vi "PPS_TRAJECTORY_EXECUTE_REL.vi"(8 "Init":bool, 10 "End Relative\nOrientation Deg":dbl, 11 "Gyro Heading\nRAD":dbl) -> (0 "AtReference":bool, 3 "Chassis Velocity Target SI":T3 {"vOmega" format="%10.3f"; "vY" format="%10.3f"; "vX" format="%10.3f"})   [LabVIEW 2019]
uses:
  <vilib>/Rock Robotics/WPI/ThirdParty/JAS_Junk/TrajLib/Trajectory_Library.lvlib
  CHS_TRAJECTORY_GLOBALS.vi
  <vilib>/Rock Robotics/WPI/ThirdParty/MJansen/PathPlanner/PathPlanner24.lvlib
  <vilib>/Rock Robotics/WPI/ThirdParty/JAS_Junk/TrajLib/TypeDef/CHASSIS_SPEEDS.ctl
  <vilib>/Rock Robotics/WPI/ThirdParty/ChoreoLib/TypeDef/ChoreoTrajectoryState.ctl
  <vilib>/Rock Robotics/WPI/ThirdParty/ChoreoLib/ChoreoLib.lvlib
  <vilib>/Rock Robotics/WPI/ThirdParty/ChoreoLib/TypeDef/ChoreoTrajectory.ctl
panel:
  out "ChoreoTrajectory":T1
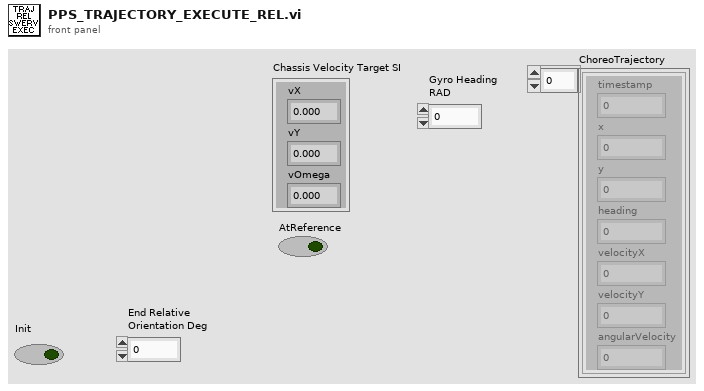
[diagram p1: front panel]
types:
  T1 = typedef "ChoreoLib.lvlib/ChoreoTrajectory.ctl" = T2[]
  T2 = typedef "ChoreoLib.lvlib/ChoreoTrajectoryState.ctl" = cluster{"timestamp":dbl, "x":dbl, "y":dbl, "heading":dbl, "velocityX":dbl, "velocityY":dbl, "angularVelocity":dbl}
  T3 = typedef "Trajectory_Library.lvlib/CHASSIS_SPEEDS.ctl" = cluster{"vX":dbl, "vY":dbl, "vOmega":dbl}
  T4 = typedef "Trajectory_Library.lvlib/SWERVE_DRIVE_KINEMATICS.ctl" = cluster{"NumModules":i32, "InverseKinematics":T5, "ForwardKinematics":T5, "Modules":T6[], "PrevCoR":T6, "SavedModuleStates":T7[]}
  T5 = typedef "NI_Matrix.lvlib/RealMatrix.ctl" = dbl[][]
  T6 = typedef "Trajectory_Library.lvlib/TRANSLATION2D.ctl" = cluster{"X":dbl, "Y":dbl}
  T7 = typedef "Trajectory_Library.lvlib/SWERVE_DRIVE_MODULE_STATE.ctl" = cluster{"Speed":dbl, "Angle":T8}
  T8 = typedef "Trajectory_Library.lvlib/ROTATION2D.ctl" = cluster{"VALUE":dbl, "COS":dbl, "SIN":dbl}
  T9 = typedef "Trajectory_Library.lvlib/SWERVE_DRIVE_MODULE_POSITION.ctl" = cluster{"Distance":dbl, "Angle":T8, "P":bool}
  T10 = typedef "Trajectory_Library.lvlib/POSE2D.ctl" = cluster{"TRANSLATION":T6, "ROTATION":T8}
  T11 = typedef "PathPlanner24.lvlib/PathPlannerTrajectoryState.ctl" = cluster{"TimeSeconds":dbl, "VelocityMPS":dbl, "AccerationMpsSq":dbl, "HeadingAngularVelRadPerSec":dbl, "PositionMeters":T6, "Heading":T8, "TargetHolonomicRotation":T8, "CurvatureRadPerMeter":dbl, "PathPlannerConstraints":T12, "DeltaPos":dbl}
  T12 = typedef "PathPlanner24.lvlib/PathPlannerPathConstraints.ctl" = cluster{"MaxVelocityMps;":dbl, "MaxAccelerationMpsSq;":dbl, "MaxAngularVelRadPsEc;":dbl, "MaxAngularAccRadPSecSq":dbl, "Exists":bool}
  T13 = typedef "Trajectory_Library.lvlib/PID_TUNING.ctl" = cluster{"Kp":dbl, "Ki":dbl, "Kd":dbl, "MaximumIntegral":dbl, "MinimumIntegral":dbl}
  T14 = typedef "Trajectory_Library.lvlib/PROFILED_PID_CONTROLLER.ctl" = cluster{"Controller":T15, "Goal":T16, "Setpoint":T16, "Constraint":T17}
  T15 = typedef "Trajectory_Library.lvlib/PID_CONTROLLER.ctl" = cluster{"Kp":dbl, "Ki":dbl, "Kd":dbl, "Period":dbl, "Max_Integral":dbl, "Min_Integral":dbl, "Max_Input":dbl, "Min_Input":dbl, "Continuous":bool, "PositionError":dbl, "VelocityError":dbl, "PrevError":dbl, "TotalError":dbl, "PositionTolerance":dbl, "VelocityTolerance":dbl, "SetPoint":dbl, "Kf":dbl, "Prev_Deriv":dbl, "Prev_Deriv 2":dbl, "DerivativeFilter":bool, "Min_Output":dbl, "Max_Output":dbl, "Prev_F_P":dbl, "Prev_F_P_2":dbl, "AntiWindupActive":bool, "Measurement":dbl}
  T16 = typedef "Trajectory_Library.lvlib/TRAPEZOID_PROFILE_STATE.ctl" = cluster{"Position":dbl, "Velocity":dbl}
  T17 = typedef "Trajectory_Library.lvlib/TRAPEZOID_PROFILE_CONSTRAINT.ctl" = cluster{"MaxVelocity":dbl, "MaxAcceleration":dbl}
  T18 = typedef "PathPlanner24.lvlib/PathPlannerCtrlHolConfig.ctl" = cluster{"HOLONOMIC_CTRL_PACK_TUNING":T19, "Max Wheel Speed M/S":dbl, "Tolerance SI":T10, "Drive Base Radius M":dbl}
  T19 = typedef "Trajectory_Library.lvlib/HOLONOMIC_PACK_TUNING.ctl" = cluster{"X PID Tuning":T13, "Y PID Tuning":T13, "thetaProfiledPID_CTRL":T14}
  T20 = typedef "Trajectory_Library.lvlib/HOLONOMIC_DRV_CTRL.ctl" = cluster{"poseTolerance":T10, "poseError":T10, "Enabled":bool, "PID_xCtrl":T15, "PID_yCtrl":T15, "PROF_PID_thetaCtrl":T14, "RotationError":T8, "FirstRun":bool}
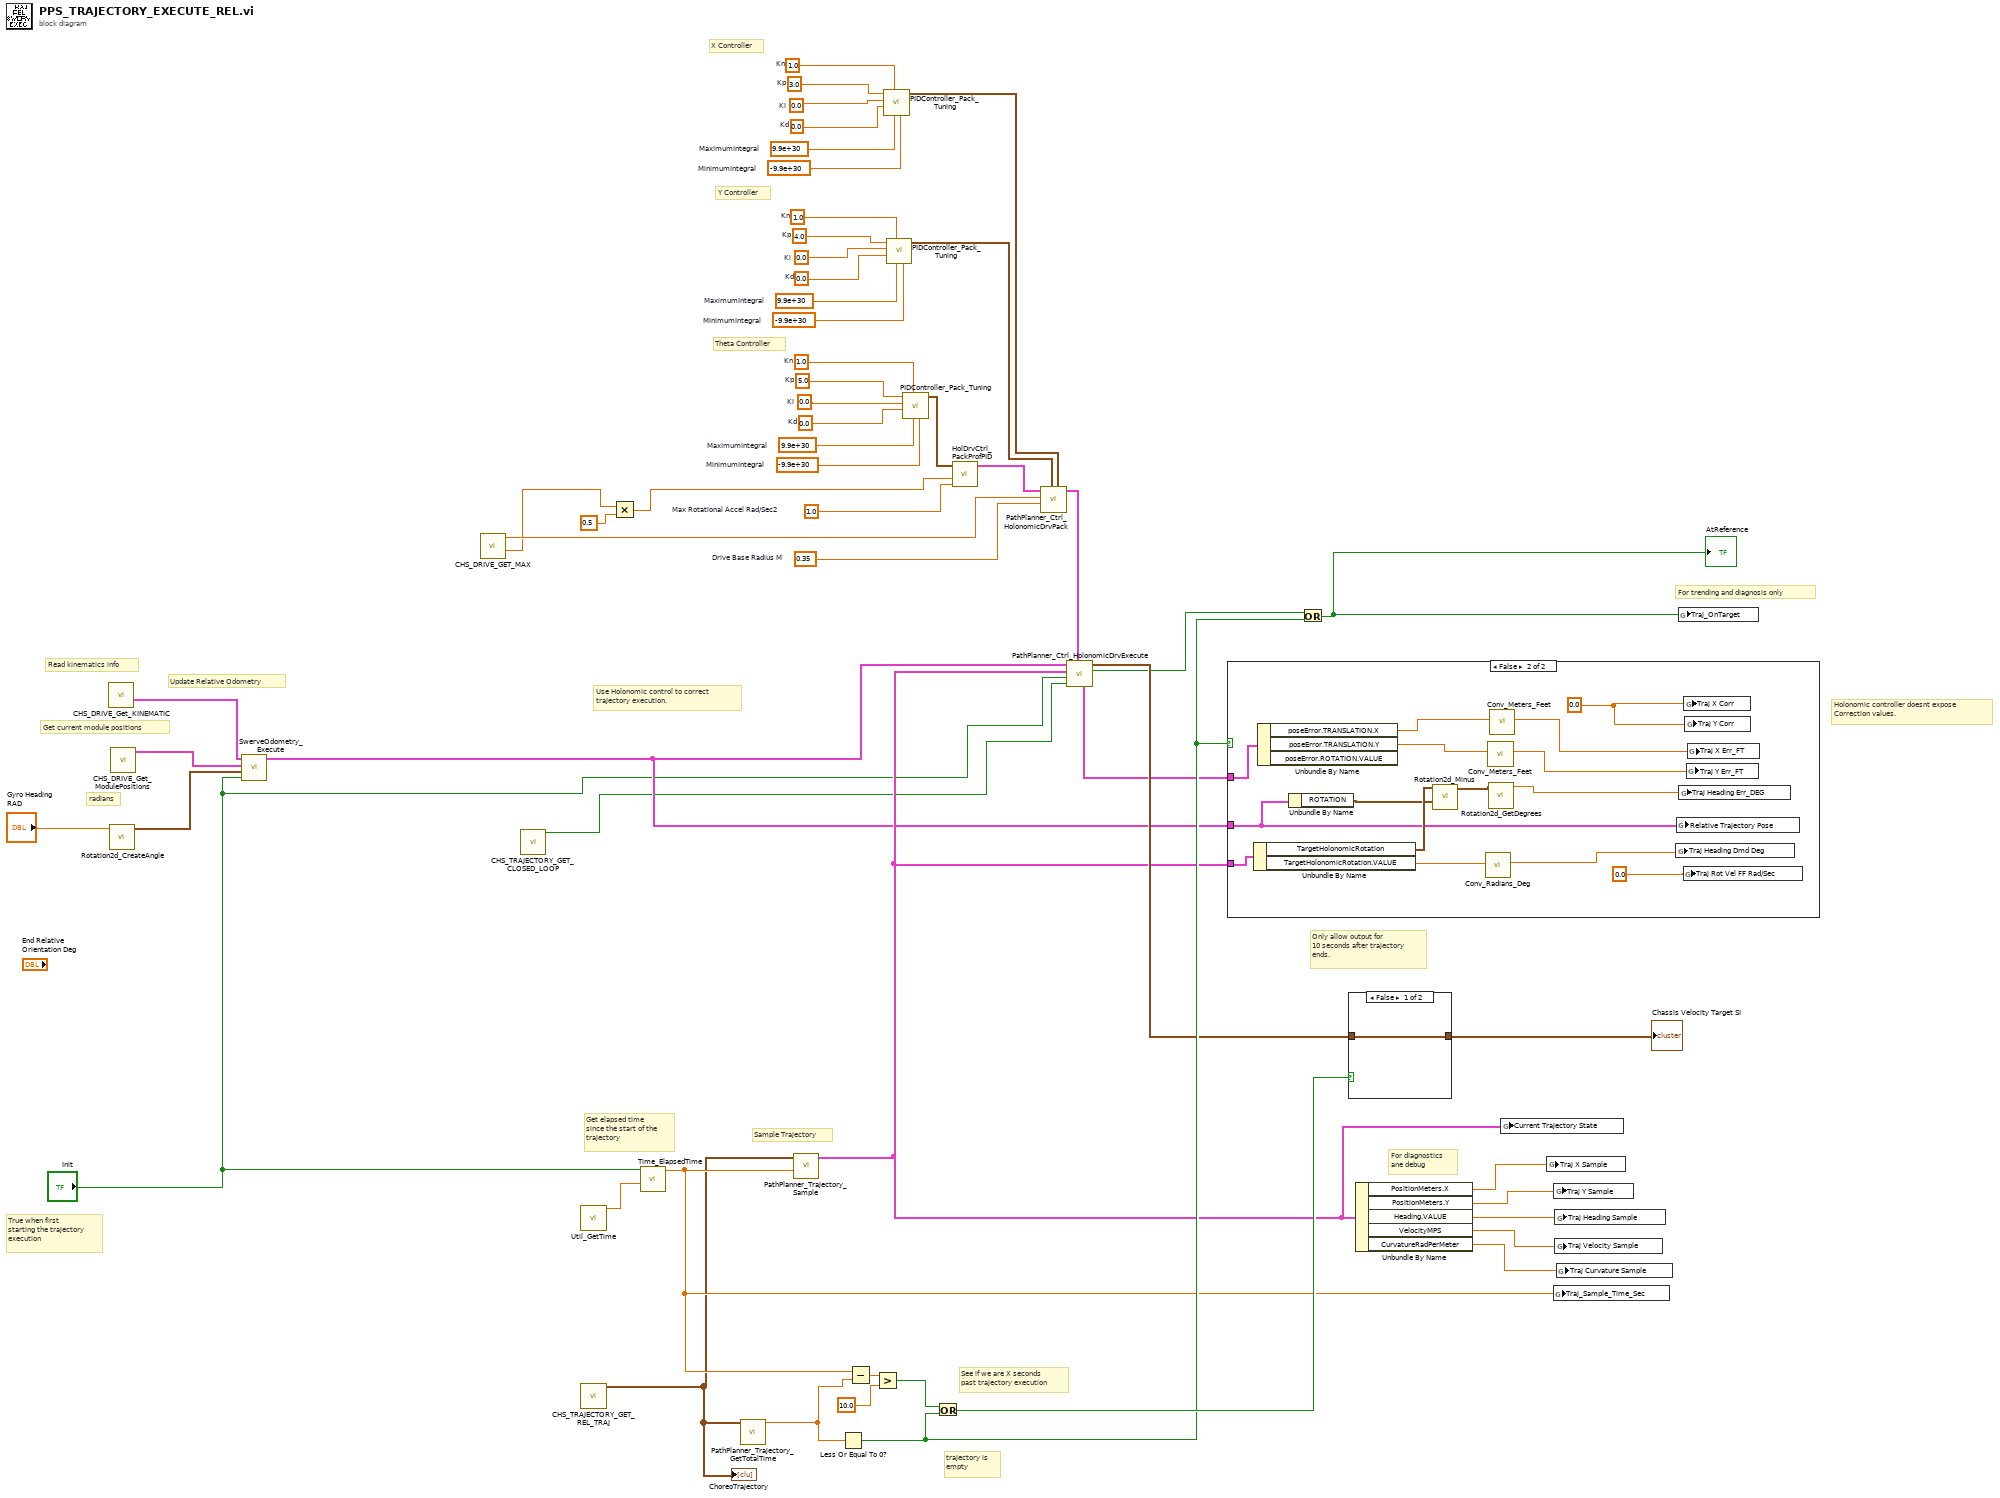
[diagram p0: block diagram]
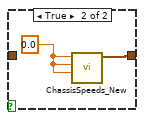
[diagram p3: hidden frame]
diagram:
  w32 = 0.35  # Drive Base Radius M
  w24 = 1.0  # Kn
  w21 = 5.0  # Kp
  w12 = 0.0  # Ki
  w11 = 0.0  # Kd
  w10 = 9.9e+30  # MaximumIntegral
  w9 = -9.9e+30  # MinimumIntegral
  w26 = 1.0  # Kn
  w23 = 3.0  # Kp
  w20 = 0.0  # Ki
  w19 = 0.0  # Kd
  w18 = 9.9e+30  # MaximumIntegral
  w17 = -9.9e+30  # MinimumIntegral
  w25 = 1.0  # Kn
  w22 = 4.0  # Kp
  w16 = 0.0  # Ki
  w15 = 0.0  # Kd
  w14 = 9.9e+30  # MaximumIntegral
  w13 = -9.9e+30  # MinimumIntegral
  w27 = 1.0  # Max Rotational Accel Rad/Sec2
  # "Theta Controller"
  # "Y Controller"
  # "X Controller"
  # "Get current module positions"
  # "Update Relative Odometry"
  # "Read kinematics info"
  # "radians"
  # "trajectory is \nempty"
  # "True when first\nstarting the trajectory\nexecution"
  # "Get elapsed time\nsince the start of the\ntrajectory"
  # "Holonomic controller doesnt expose\nCorrection values."
  # "Use Holonomic control to correct\ntrajectory execution."
  # "For trending and diagnosis only"
  # "For diagnostics\nane debug"
  # "Sample Trajectory"
  # "See if we are X seconds \npast trajectory execution"
  # "Only allow output for\n10 seconds after trajectory\nends."
  n1 = call "CHS_DRIVE_Get_KINEMATIC.vi"() -> ("out SWERVE_DRIVE_KINEMATICS"=w35:T4)  [unwired: 11 in]
  n2 = call <vilib>:"Rotation2d_CreateAngle.vi"("Angle"="Gyro Heading\nRAD") -> ("ROTATION"=w37:T8)  [unwired: 10 in]
  n3 = call "CHS_DRIVE_Get_ModulePositions.vi"() -> ("Swerve Module Positions"=w36:T9[])  [unwired: 11 in]
  n4 = call <vilib>:"SwerveOdometry_Execute.vi"("Init"="Init", "Rotation"=w37, "Swerve Module Positions"=w36, "SWERVE_DRIVE_KINEMATICS"=w35) -> ("Current Pose"=w34:T10)  [unwired: 5 in, 2 out]
  n5 = call "CHS_DRIVE_GET_MAX.vi"() -> ("Max Rotational Vel (Rad/Sec)"=w2:dbl, "Max Wheel Vel (Meter/Sec)"=w6:dbl)  [unwired: 10 in]
  n6 = call "CHS_TRAJECTORY_GET_CLOSED_LOOP.vi"() -> ("AUTO_CLOSED_LOOP"=w4:bool)  [unwired: 11 in]
  n7 = call <vilib>:"Util_GetTime.vi"() -> ("FPGA_Time_Seconds"=w53:dbl)  [unwired: 9 in, 2 out]
  n8 = call "CHS_TRAJECTORY_GET_REL_TRAJ.vi"() -> ("Relative_Trajectory"=w38:T1)  [unwired: 11 in]
  "ChoreoTrajectory" <- w38
  n9 = Multiply(x=w2, y=0.5) -> (x*y=w1:dbl)
  n10 = call <vilib>:"Time_ElapsedTime.vi"("PassthroughTime_SEC"=w53, "Reset"="Init") -> ("Elapsed Time Sec"=w43:dbl)  [unwired: 9 in]
  n11 = call <vilib>:"PathPlanner_Trajectory_GetTotalTime.vi"("PathPlannerTrajectory"=w38) -> ("TotalTimeSeconds"=w40:dbl)  [unwired: 10 in]
  n12 = call <vilib>:"PathPlanner_Trajectory_Sample.vi"("Time"=w43, "PathPlannerTrajectory"=w38) -> ("PathPlannerState"=w39:T11)  [unwired: 9 in]
  n13 = Less Or Equal To 0?(x=w40) -> (x <= 0?=w44:bool)
  n14 = Subtract(x=w43, y=w40) -> (x-y=w56:dbl)
  n15 = Greater?(x=w56, y=10.0) -> (0:w47:bool)
  n16 = call <vilib>:"PIDController_Pack_Tuning.vi"("MinimumIntegral"=w17, "MaximumIntegral"=w18, "Kn"=w26, "Kd"=w19, "Ki"=w20, "Kp"=w23) -> ("PID Tuning"=w29:T13)  [unwired: 5 in]
  n17 = call <vilib>:"PIDController_Pack_Tuning.vi"("MinimumIntegral"=w13, "MaximumIntegral"=w14, "Kn"=w25, "Kd"=w15, "Ki"=w16, "Kp"=w22) -> ("PID Tuning"=w30:T13)  [unwired: 5 in]
  n18 = call <vilib>:"PIDController_Pack_Tuning.vi"("MinimumIntegral"=w9, "MaximumIntegral"=w10, "Kn"=w24, "Kd"=w11, "Ki"=w12, "Kp"=w21) -> ("PID Tuning"=w28:T13)  [unwired: 5 in]
  n19 = Or(x=w47, y=w44) -> (x .or. y?=w46:bool)
  n20 = call <vilib>:"HolDrvCtrl_PackProfPID.vi"("Max Accel"=w27, "Max Speed"=w1, "Theta PID Tuning"=w28) -> ("Theta PID CONTROLLER"=w31:T14)  [unwired: 8 in]
  n21 = call <vilib>:"PathPlanner_Ctrl_HolonomicDrvPack.vi"("X PID Tuning"=w29, "Y PID Tuning"=w30, "Drive Base Radius M"=w32, "Max Wheel Speed M/S"=w6, "thetaProfiledPID_CTRL"=w31) -> ("PathPlanner_Ctrl_HolDrvConfig"=w8:T18)  [unwired: 6 in]
  n22 = call <vilib>:"PathPlanner_Ctrl_HolonomicDrvExecute.vi"("PathPlanner_Ctrl_HolDrvConfig"=w8, "Enabled"=w4, "Reset"="Init", "PathPlannerState"=w39, "Current Pose SI"=w34) -> ("At Reference"=w41:bool, "calcChassisSpeed"=w42:T3, "outHOLONOMIC_DRV_CTRL"=w7:T20)  [unwired: 3 in, 1 out]
  n23 = case shown="False" w44 {
    tunnel: w34 -> [_ w60]
    tunnel: w7 -> [_ w67]
    tunnel: w39 -> [_ w64]
    frame True {
    }
    frame False {
      w71 = 0.0 ("Y Corr")
      n24 = Unbundle By Name(w64) -> ("TargetHolonomicRotation"=w61:T8, "TargetHolonomicRotation.VALUE"=w63:dbl)
      n25 = Unbundle By Name(w67) -> ("poseError.TRANSLATION.X"=w66:dbl, "poseError.TRANSLATION.Y"=w65:dbl)  [unwired: 1 out]
      n26 = Unbundle By Name(w60) -> ("ROTATION"=w59:T8)
      n27 = call <vilib>:"Rotation2d_Minus.vi"("other ROTATION"=w59, "in ROTATION"=w61) -> ("out ROTATION"=w58:T8)  [unwired: 9 in]
      n28 = call <vilib>:"Conv_Radians_Deg.vi"("Radians"=w63) -> ("Degrees"=w62:dbl)  [unwired: 10 in]
      n29 = call <vilib>:"Conv_Meters_Feet.vi"("Meters"=w65) -> ("Feet"=w70:dbl)  [unwired: 10 in]
      n30 = call <vilib>:"Rotation2d_GetDegrees.vi"("in ROTATION"=w58) -> ("AngleDegrees"=w57:dbl)  [unwired: 10 in]
      n31 = call <vilib>:"Conv_Meters_Feet.vi"("Meters"=w66) -> ("Feet"=w69:dbl)  [unwired: 10 in]
      n32 = global write "CHS_TRAJECTORY_GLOBALS.vi" "Traj Heading Dmd Deg"(w62) -> ()
      n33 = global write "CHS_TRAJECTORY_GLOBALS.vi" "Relative Trajectory Pose"(w60) -> ()
      n34 = global write "CHS_TRAJECTORY_GLOBALS.vi" "Traj Heading Err_DEG"(w57) -> ()
      n35 = global write "CHS_TRAJECTORY_GLOBALS.vi" "Traj Rot Vel FF Rad/Sec"(0.0 ("Traj Heading Dmd Deg")) -> ()
      n36 = global write "CHS_TRAJECTORY_GLOBALS.vi" "Traj X Corr"(w71) -> ()
      n37 = global write "CHS_TRAJECTORY_GLOBALS.vi" "Traj Y Corr"(w71) -> ()
      n38 = global write "CHS_TRAJECTORY_GLOBALS.vi" "Traj Y Err_FT"(w70) -> ()
      n39 = global write "CHS_TRAJECTORY_GLOBALS.vi" "Traj X Err_FT"(w69) -> ()
    }
  }
  n40 = Or(x=w41, y=w44) -> (x .or. y?=w45:bool)
  "AtReference" <- w45
  n41 = case shown="False" w46 {
    tunnel: w42 -> [w72 _]
    tunnel: [w72 w73] -> w54
    frame False {
    }
    frame True {
      w74 = 0.0 ("vX")
      n42 = call <vilib>:"ChassisSpeeds_New.vi"("vAngular"=w74, "vY"=w74, "vX"=w74) -> ("CHASSIS"=w73:T3)  [unwired: 8 in]
    }
  }
  "Chassis Velocity Target SI" <- w54
  n43 = Unbundle By Name(w39) -> ("PositionMeters.X"=w52:dbl, "PositionMeters.Y"=w51:dbl, "Heading.VALUE"=w50:dbl, "VelocityMPS"=w49:dbl, "CurvatureRadPerMeter"=w48:dbl)
  n44 = global write "CHS_TRAJECTORY_GLOBALS.vi" "Current Trajectory State"(w39) -> ()
  n45 = global write "CHS_TRAJECTORY_GLOBALS.vi" "Traj X Sample"(w52) -> ()
  n46 = global write "CHS_TRAJECTORY_GLOBALS.vi" "Traj_Sample_Time_Sec"(w43) -> ()
  n47 = global write "CHS_TRAJECTORY_GLOBALS.vi" "Traj Y Sample"(w51) -> ()
  n48 = global write "CHS_TRAJECTORY_GLOBALS.vi" "Traj Heading Sample"(w50) -> ()
  n49 = global write "CHS_TRAJECTORY_GLOBALS.vi" "Traj Velocity Sample"(w49) -> ()
  n50 = global write "CHS_TRAJECTORY_GLOBALS.vi" "Traj Curvature Sample"(w48) -> ()
  n51 = global write "CHS_TRAJECTORY_GLOBALS.vi" "Traj_OnTarget"(w45) -> ()
